vi "sub_ofdm_delayed_mult_CFO_sync_single.vi"(8 "CP length":i32=64, 9 "FFT size":i32=256, 11 "time samples":cdb[](array[numeric])) -> (3 "sync ofdm symbol":cdb[](array[numeric]))   [LabVIEW 2014]
uses:
  <vilib>/Analysis/1siggen.llb/Ramp Pattern by Samples.vi
  <vilib>/Analysis/NI_AALBase.lvlib
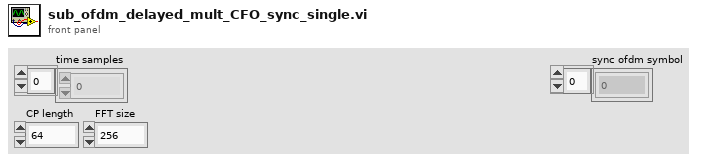
[diagram p1: front panel]
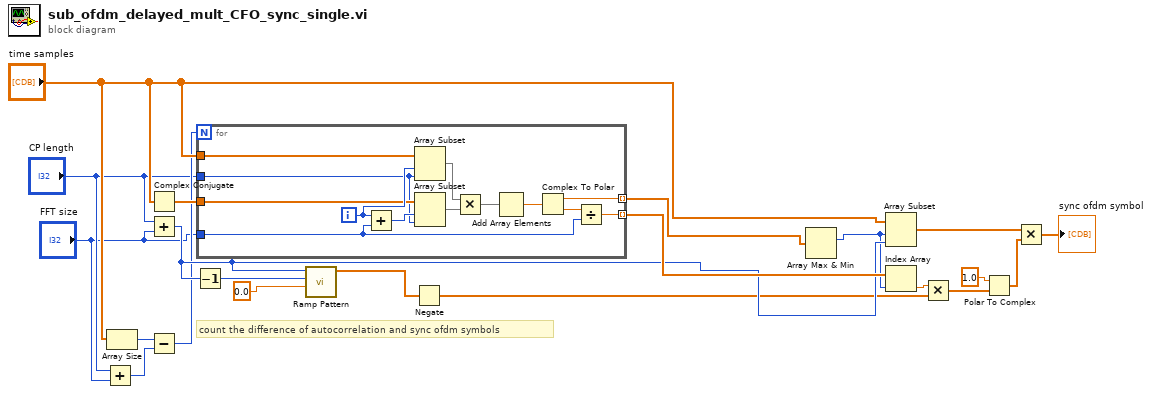
[diagram p0: block diagram]
diagram:
  # "count the difference of autocorrelation and sync ofdm symbols"
  n1 = Add(x="CP length", y="FFT size") -> (x+y=w10:i32)
  n2 = Array Size(array="time samples") -> (size(s)=w9:i32)
  n3 = Complex Conjugate(1:"time samples") -> (0:w21:cdb[])
  n4 = Add(x="CP length", y="FFT size") -> (x+y=w18:i32)
  n5 = Subtract(x=w9, y=w10) -> (x-y=w13:i32)
  n6 = Decrement(x=w18) -> (x-1=w17:i32)
  n7 = for {
    N: w13 -> [_]
    tunnel: "time samples" -> [w34]
    tunnel: w21 -> [w32]
    tunnel: "FFT size" -> [w22]
    tunnel: [w26] -> w20 mode=indexing
    tunnel: [w24] -> w3 mode=indexing
    tunnel: "CP length" -> [w23]
    i -> [w33]
    n8 = Add(x=w33, y=w22) -> (x+y=w31:i32)
    n9 = Array Subset(array=w34, index=w33, length=w23) -> (w29:cdb[])
    n10 = Array Subset(array=w32, index=w31, length=w23) -> (w30:cdb[])
    n11 = Multiply(x=w29, y=w30) -> (x*y=w28:cdb[])
    n12 = Add Array Elements(numeric array=w28) -> (sum=w25:cdb)
    n13 = Complex To Polar(r * e^(i*theta)=w25) -> (r=w24:dbl, theta=w27:dbl)
    n14 = Divide(x=w27, y=w22) -> (x/y=w26:dbl)
  }
  n15 = call-poly <vilib>:"Ramp Pattern.vi"("start"=0.0, "end"=w17, "samples"=w18) -> ("Ramp Pattern"=w15:dbl[])  [unwired: 7 in, 1 out]
  n16 = Negate(x=w15) -> (-x=w14:dbl[])
  n17 = Array Max & Min(array=w3) -> (max index (indices)=w2:i32)  [unwired: 3 out]
  n18 = Array Subset(array="time samples", index=w2, length=w18) -> (w4:cdb[])
  n19 = Index Array(array=w20, index=w2) -> (element=w5:dbl)
  n20 = Multiply(x=w5, y=w14) -> (x*y=w7:dbl[])
  n21 = Polar To Complex(1:w7, 2:1.0) -> (0:w6:cdb[])
  n22 = Multiply(x=w4, y=w6) -> (x*y=→"sync ofdm symbol":cdb[])
